vi "MultilineBuffer.vi"(6 "Buffer Size":i32, 9 "Buffer In":string[](array[string]), 10 "New Flag":bool, 11 "Line In":string) -> (3 "Buffer Out":string[](array[string]))   [LabVIEW 2015]
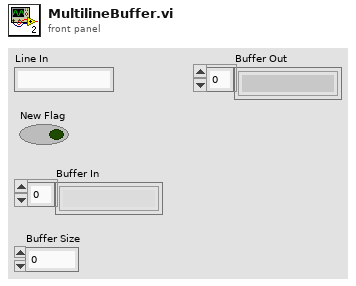
[diagram p1: front panel]
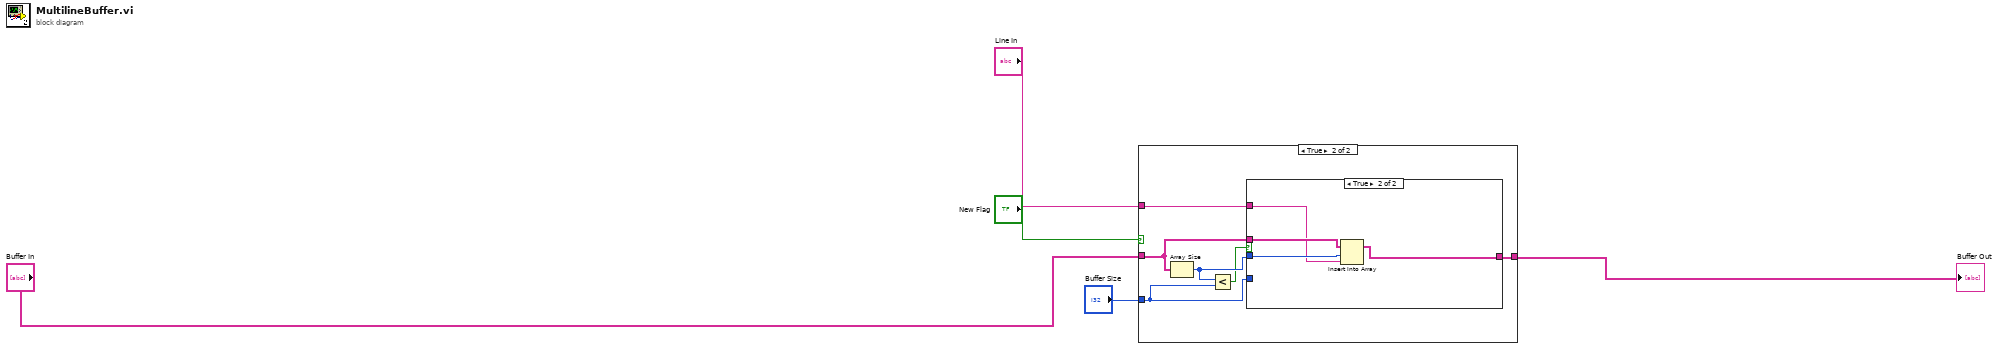
[diagram p0: block diagram]
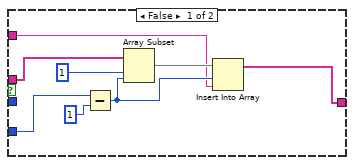
[diagram p3: hidden frame]
diagram:
  n1 = case shown="True" "New Flag" {
    tunnel: "Line In" -> [_ w10]
    tunnel: [w6 w9] -> w2
    tunnel: "Buffer In" -> [w6 w8]
    tunnel: "Buffer Size" -> [_ w7]
    frame False {
    }
    frame True {
      n2 = Array Size(array=w8) -> (size(s)=w12:i32)
      n3 = Less?(x=w12, y=w7) -> (x < y?=w11:bool)
      n4 = case shown="True" w11 {
        tunnel: w8 -> [w20 w24]
        tunnel: w12 -> [_ w23]
        tunnel: [w14 w22] -> w9
        tunnel: w7 -> [w18 _]
        tunnel: w10 -> [w13 w21]
        frame False {
          n5 = Subtract(x=w18, y=1) -> (x-y=w15:i32)
          n6 = Array Subset(array=w20, index=1, length=w15) -> (w16:string[])
          n7 = Insert Into Array(array=w16, index=w15, new element=w13) -> (w14:string[])
        }
        frame True {
          n8 = Insert Into Array(array=w24, index=w23, new element=w21) -> (w22:string[])
        }
      }
    }
  }
  "Buffer Out" <- w2
